vi "Set Enable State on Multiple Controls.vi"(8 "error in (no error)":errorcluster, 9 "Enable?":bool, 11 "Controls":refnum<vi>[](array[refnum])) -> (0 "error out":errorcluster)   [LabVIEW 2014]
doc: "Sets all the controls in the input array to the \"Enable state\" value."
panel:
  # "LICENSED MATERIALS – PROPERTY OF IBM\nCopyright IBM Corp. 2016,\nALL RIGHTS RESERVED"
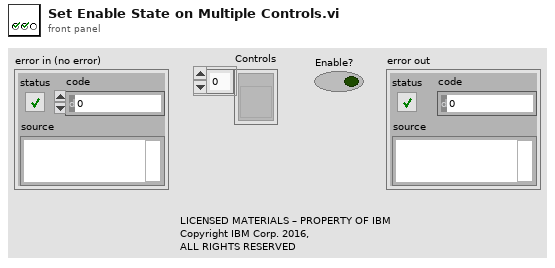
[diagram p1: front panel]
types:
  T1 = enum8{"Enabled", "Disabled", "Disabled and Grayed Out"}
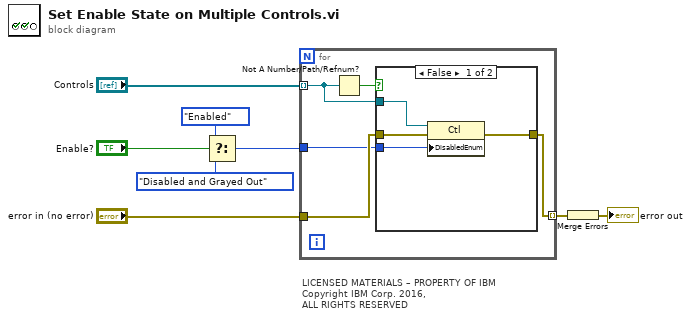
[diagram p0: block diagram]
diagram:
  # "LICENSED MATERIALS – PROPERTY OF IBM\nCopyright IBM Corp. 2016,\nALL RIGHTS RESERVED"
  n1 = Select(t=T1."Enabled" ("Enabled"), s="Enable?", f=T1."Disabled and Grayed Out" ("Disabled")) -> (s? t:f=w1:T1)
  n2 = for {
    tunnel: "Controls" -> [w12] mode=indexing
    tunnel: "error in (no error)" -> [w11]
    tunnel: [w10] -> w6 mode=indexing
    tunnel: w1 -> [w9]
    n3 = Not A Number/Path/Refnum?(number/path/refnum=w12) -> (NaN/Path/Refnum?=w13:bool)
    n4 = case shown="False" w13 {
      tunnel: w12 -> [w17 _]
      tunnel: w11 -> [w16 w18]
      tunnel: [w15 w18] -> w10
      tunnel: w9 -> [w14 _]
      frame False {
        n5 = property class="Ctl"(reference=w17, error in=w16, "DisabledEnum"=w14) -> (error out=w15:errorcluster)  [unwired: 1 out]
      }
      frame True {
      }
    }
  }
  n6 = Merge Errors(w6) -> (→"error out":errorcluster)
